vi "source_parameter_strict_type_to_strings.vi"(8 "error in (no error)":errorcluster, 10 "Source parameters":T1) -> (0 "error out":errorcluster, 2 "Source parameters (strings)":T2)   [LabVIEW 2018]
uses:
  source_parameters_strings.ctl
  source_parameters.ctl
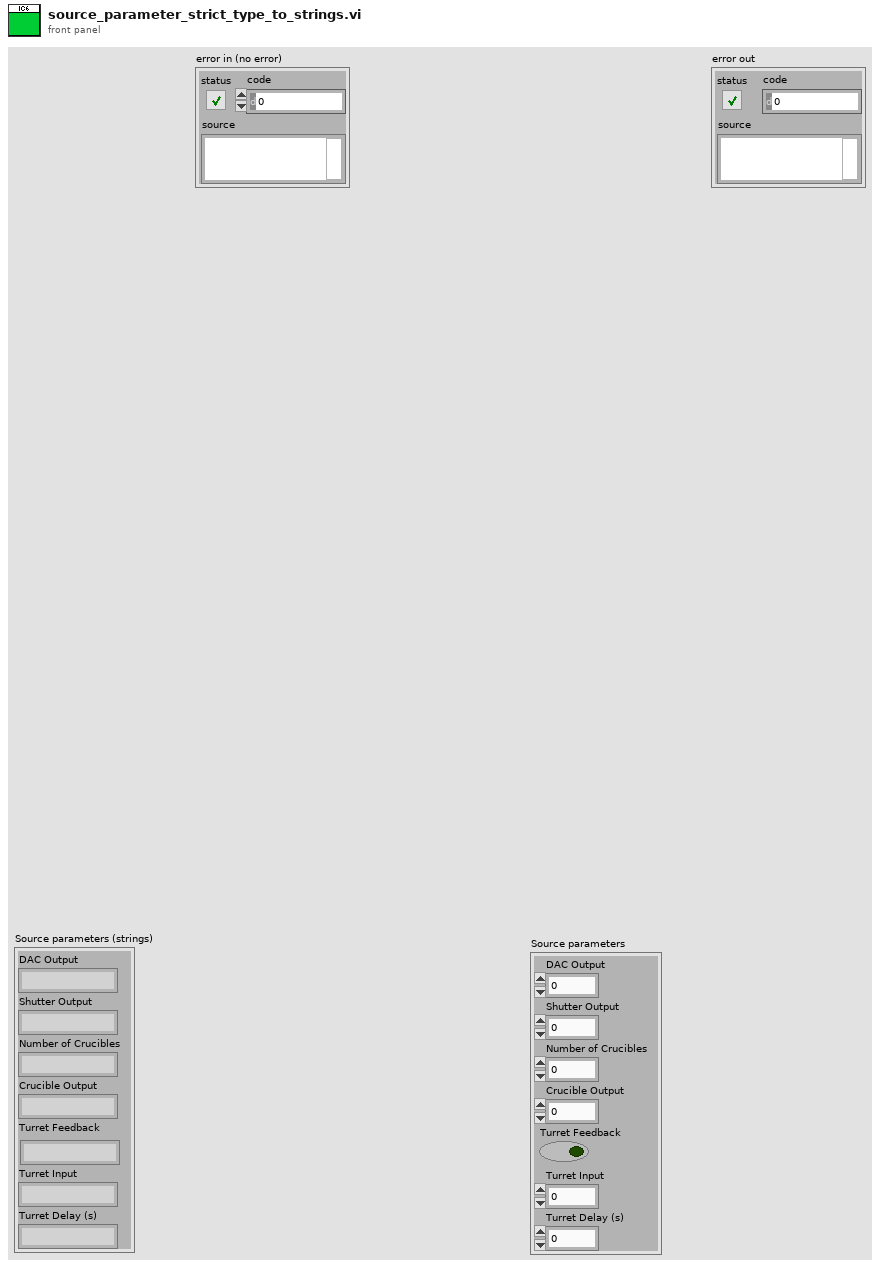
[diagram p1: front panel]
types:
  T1 = typedef "source_parameters.ctl" = cluster{"DAC Output":u8, "Shutter Output":u8, "Number of Crucibles":u8, "Crucible Output":u8, "Turret Feedback":bool, "Turret Input":u8, "Turret Delay (s)":u8}
  T2 = typedef "source_parameters_strings.ctl" = cluster{"DAC Output":string, "Shutter Output":string, "Number of Crucibles":string, "Crucible Output":string, "Turret Feedback":string, "Turret Input":string, "Turret Delay (s)":string}
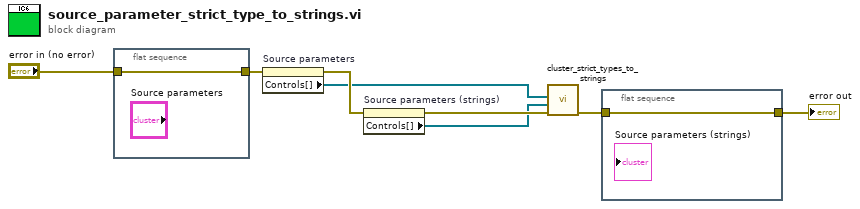
[diagram p0: block diagram]
diagram:
  n1 = flat-sequence {
    tunnel: "error in (no error)" -> [w9]
    tunnel: [w9] -> w6
    frame #0 {
    }
  }
  n2 = property on="Source parameters" class="Clust (strict)"(error in=w6) -> (error out=w5:errorcluster, "Controls[]"=w3:refnum<vi>[])  [unwired: 1 in, 1 out]
  n3 = property on="Source parameters (strings)" class="Clust (strict)"(error in=w5) -> (error out=w4:errorcluster, "Controls[]"=w2:refnum<vi>[])  [unwired: 1 in, 1 out]
  n4 = call "cluster_strict_types_to_strings.vi"("error in (no error)"=w4, "Controls[] (strings)"=w2, "Controls[]"=w3) -> ("error out"=w1:errorcluster)  [unwired: 8 in]
  n5 = flat-sequence {
    tunnel: w1 -> [w10]
    tunnel: [w10] -> w7
    frame #0 {
    }
  }
  "error out" <- w7
